vi "Create Message Data Cluster.vi"(6 "generate serialization helpers":bool, 7 "owning typedef":refnum<vi>, 8 "error in (no error)":errorcluster, 9 "library in":refnum<vi>, 10 "message element metafata":T1[](array[typedef]), 11 "cluster in":refnum<vi>) -> (0 "error out":errorcluster, 1 "library out":refnum<vi>, 3 "cluster out":refnum<vi>)   [LabVIEW 2019, in "gRPC Template Creation Utility.lvlib"]
uses:
  gRPC Template Creation Utility.lvlib
  <vilib>/Utility/miscctls.llb/LVPositionTypeDef.ctl
  TypeDefs/Message Element Type.ctl
  TypeDefs/Message Element Metadata (Scripting).ctl
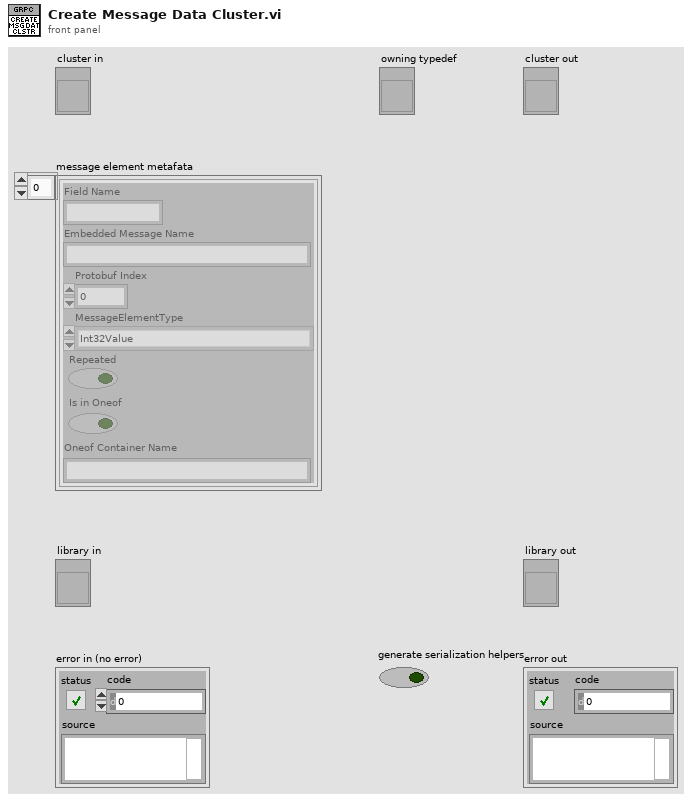
[diagram p1: front panel]
types:
  T1 = typedef "gRPC Template Creation Utility.lvlib/Message Element Metadata (Scripting).ctl" = cluster{"Field Name":string, "Embedded Message Name":string, "Protobuf Index":i32, "MessageElementType":T2, "Repeated":bool, "Is in Oneof":bool, "Oneof Container Name":string}
  T2 = typedef "gRPC Template Creation Utility.lvlib/Message Element Type.ctl" = enum32{"Int32Value", "FloatValue", "DoubleValue", "BoolValue", "StringValue", "MessageValue", "Int64Value", "UInt32Value", "UInt64Value", "EnumValue", "Bytes", "Fixed64", "Fixed32", "SFixed64", "SFixed32", "SInt64", "SInt32"}
  T3 = typedef "LVPositionTypeDef.ctl" = cluster{"Left":i32, "Top":i32}
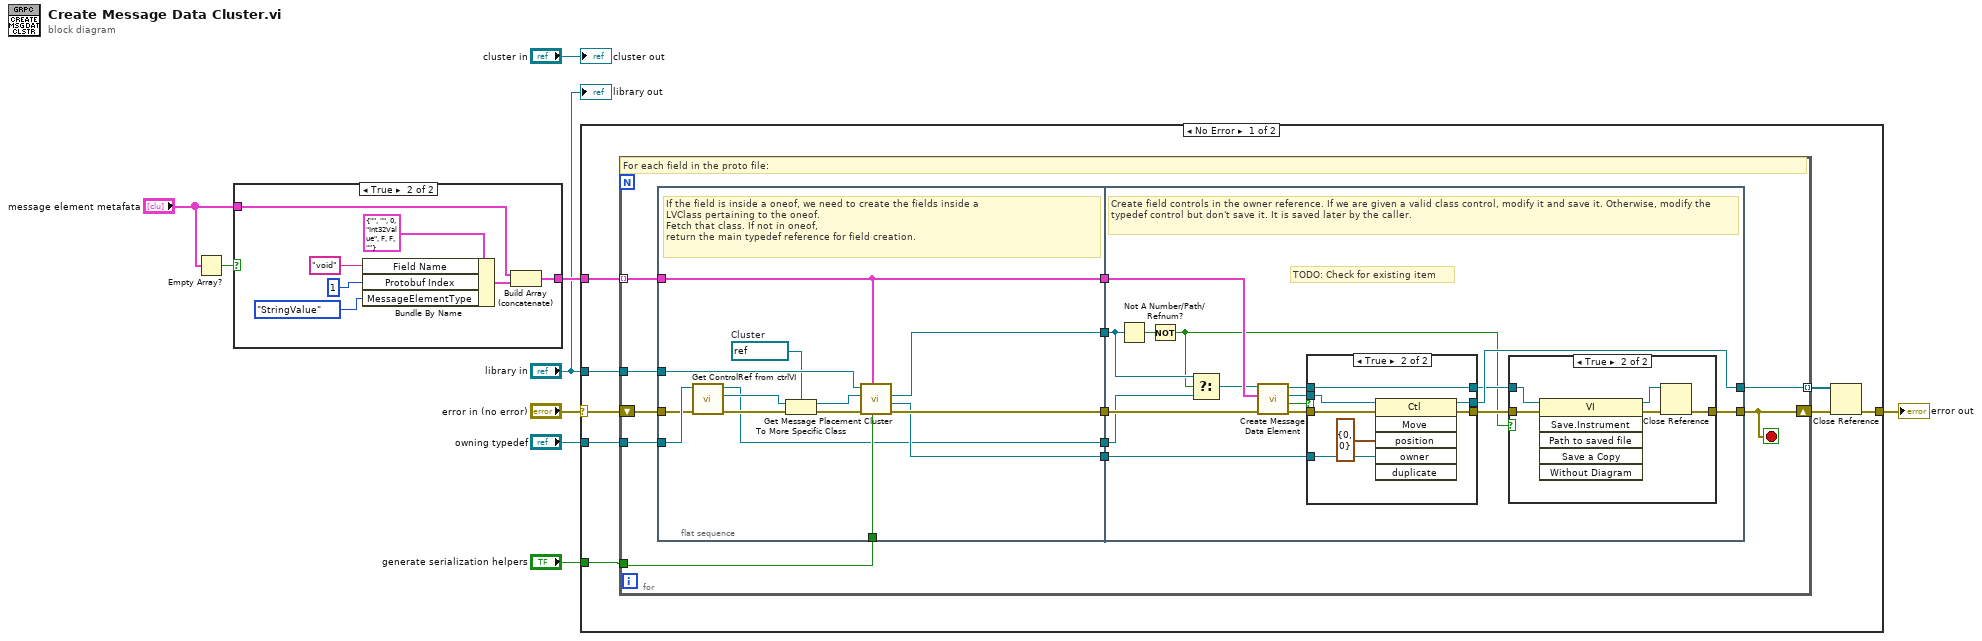
[diagram p0: block diagram]
diagram:
  n1 = Empty Array?(array="message element metafata") -> (empty?=w6:bool)
  n2 = case shown="True" w6 {
    tunnel: "message element metafata" -> [w10 w17]
    tunnel: [w10 w16] -> w5
    frame False {
    }
    frame True {
      n3 = Bundle By Name(cluster=T1 {"Field Name"="", "Embedded Message Name"="", "Protobuf Index"=0, "MessageElementType"=enum."Int32Value", "Repeated"=FALSE, "Is in Oneof"=FALSE, "Oneof Container Name"=""} ("MessageElementMetadata"), "Field Name"="void", "Protobuf Index"=1, "MessageElementType"=Message_Element_Type."StringValue") -> (w11:T1)
      n4 = Build Array (concatenate)(w17, w11) -> (w16:T1[])
    }
  }
  n5 = case shown="No Error" "error in (no error)" {
    selector: "error in (no error)" -> [w21 w84]
    tunnel: [w19 w84] -> w9
    tunnel: "library in" -> [w23 _]
    tunnel: w5 -> [w22 _]
    tunnel: "generate serialization helpers" -> [w20 _]
    tunnel: "owning typedef" -> [w18 _]
    frame No Error {
      n6 = for {
        tunnel: [w33] -> w25 mode=indexing
        shift-right: [w29] -> w24
        shift-left: w21 -> [w37]
        tunnel: w22 -> [w34] mode=indexing
        tunnel: w23 -> [w36]
        tunnel: w20 -> [w32]
        tunnel: w18 -> [w27]
        stop <- w29 stop-if-true
        # "For each field in the proto file:"
        n7 = flat-sequence {
          tunnel: w34 -> [w47]
          tunnel: w37 -> [w40]
          tunnel: w36 -> [w49]
          tunnel: [w51] -> w35
          tunnel: w32 -> [w50]
          tunnel: [w48] -> w31
          tunnel: [w47] -> w30
          tunnel: [w41] -> w28
          tunnel: w27 -> [w46]
          tunnel: [w38] -> w26
          tunnel: w35 -> [w67]
          tunnel: w31 -> [w66]
          tunnel: w30 -> [w61]
          tunnel: [w65] -> w33
          tunnel: [w54] -> w29
          tunnel: w28 -> [w59]
          tunnel: w26 -> [w52]
          frame #0 {
            w45 = refnum<vi> refnum  # Cluster
            # "If the field is inside a oneof, we need to create the fields inside a \nLVClass pertaining to the oneof. \nFetch that class. If not in oneof, \nreturn the main typedef reference for field creation."
            n8 = call "Get ControlRef from ctrlVI.vi"("error in (no error)"=w40, "VI ref in"=w46) -> ("error out"=w43:errorcluster, "Control ref out"=w44:refnum<vi>, "VI ref out"=w38:refnum<vi>)  [unwired: 7 in]
            n9 = To More Specific Class(target class=w45, reference=w44, error in=w43) -> (specific class reference=w42:refnum<vi>, error out=w39:errorcluster)
            n10 = call "Get Message Placement Cluster.vi"("Is Serialization Cluster"=w50, "MessageElementMetadata"=w47, "error in (no error)"=w39, "typedef cluster"=w42, "library in"=w49) -> ("error out"=w51:errorcluster, "owning cluster"=w48:refnum<vi>, "class data control"=w41:refnum<vi>)  [unwired: 3 in, 1 out]
          }
          frame #1 {
            # "TODO: Check for existing item"
            # "Create field controls in the owner reference. If we are given a valid class control, modify it and save it. Otherwise, modify the typedef control but don't save it. It is saved later by the caller."
            n11 = Not A Number/Path/Refnum?(number/path/refnum=w59) -> (NaN/Path/Refnum?=w60:bool)
            n12 = Not(x=w60) -> (.not. x?=w53:bool)
            n13 = Select(t=w59, s=w53, f=w52) -> (s? t:f=w58:refnum<vi>)
            n14 = call "Create Message Data Element.vi"("error in (no error)"=w67, "message element metadata"=w61, "owning vi in"=w58) -> ("error out"=w62:errorcluster, "data element created"=w64:bool, "data element control"=w63:refnum<vi>, "owning vi out"=w57:refnum<vi>)  [unwired: 5 in]
            n15 = case shown="True" w64 {
              tunnel: w66 -> [_ w83]
              tunnel: [w76 w82] -> w65
              tunnel: w63 -> [w76 w80]
              tunnel: w62 -> [w75 w79]
              tunnel: [w75 w78] -> w56
              tunnel: w57 -> [w74 w77]
              tunnel: [w74 w77] -> w55
              frame False {
              }
              frame True {
                n16 = invoke class="Ctl" method="Move"(reference=w80, error in=w79, "position"=T3 {"Left"=0, "Top"=0}, "owner"=w83) -> (reference out=w82:refnum<vi>, error out=w78:errorcluster)  [unwired: 2 in, 4 out]
              }
            }
            n17 = case shown="True" w53 {
              tunnel: w56 -> [w68 w72]
              tunnel: w55 -> [_ w73]
              tunnel: [w68 w70] -> w54
              frame False {
              }
              frame True {
                n18 = invoke class="VI" method="Save.Instrument"(reference=w73, error in=w72) -> (reference out=w69:refnum<vi>, error out=w71:errorcluster)  [unwired: 4 in, 4 out]
                n19 = Close Reference(reference=w69, error in (no error)=w71) -> (error out=w70:errorcluster)
              }
            }
          }
        }
      }
      n20 = Close Reference(reference=w25, error in (no error)=w24) -> (error out=w19:errorcluster)
    }
    frame Error {
    }
  }
  "error out" <- w9
  "cluster out" <- "cluster in"
  "library out" <- "library in"
